vi "Test Summary on Failing Case Result.vi"(8 "error in (no error)":errorcluster, 11 "Result Model Result Recording Test in":refnum<class "Result Model Result Recording Test.lvclass">) -> (0 "error out":errorcluster, 3 "Result Model Result Recording Test out":refnum<class "Result Model Result Recording Test.lvclass">)   [LabVIEW 2020, in "Result Model Result Recording Test.lvclass"]
uses:
  Result Model Result Recording Test.lvclass
  Result Model Result Recording Test.lvclass/Result Model Result Recording Test.ctl
  source/Core/Result/Type.ctl
  source/Core/Result/Result.lvlib
  source/Core/Result/Status.ctl
  source/Core/Result/Result.ctl
  source/User Interface/Result Model/Result Model.lvclass
  ae2c71b8-32bb-49d1-8500-0119bfec74ff.vi
  C:/git/astemes-lunit/source/User Interface/Result Model/Result Model.lvclass
  C:/git/astemes-lunit/source/Framework/Result Observer/Result Observer.lvclass
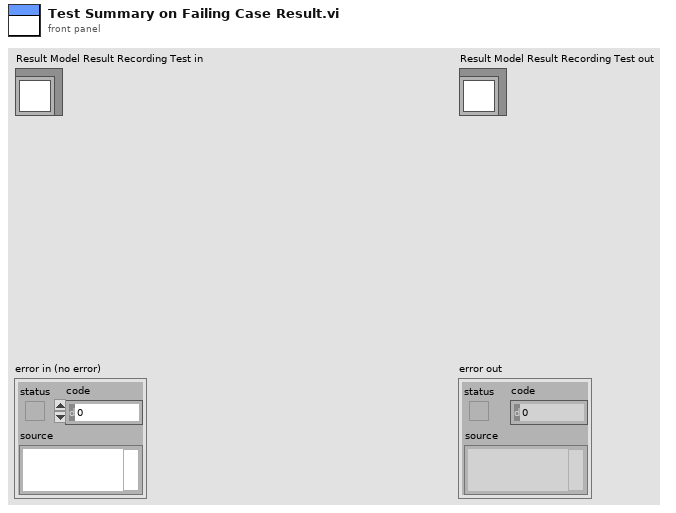
[diagram p1: front panel]
types:
  T1 = typedef "Result.lvlib/Result.ctl" = cluster{"Name":string, "Message":string, "Description":string, "Status":T2, "Result Type":T3, "Execution Time":dbl}
  T2 = typedef "Result.lvlib/Status.ctl" = enum16{"", "Passed", "Failed", "Error", "Skipped", "Setup Error", "Broken", "Teardown Error"}
  T3 = typedef "Result.lvlib/Type.ctl" = enum16{"Method", "Case", "Suite", "Pass", "Fail", "Skip", "Pass if", "Fail if", "Pass if Error", "Fail if Error", "Pass if Equal", "Fail if Equal"}
  T4 = cluster{"Left Cell String":string, "Child Text":string[], "Child Tag":string, "Item Indent":i32, "Child Only?":bool, "Glyph Index":i32}[]
  T5 = cluster{"Left Cell String":string, "Child Text":string[], "Child Tag":string, "Item Indent":i32, "Child Only?":bool, "Glyph Index":i32}
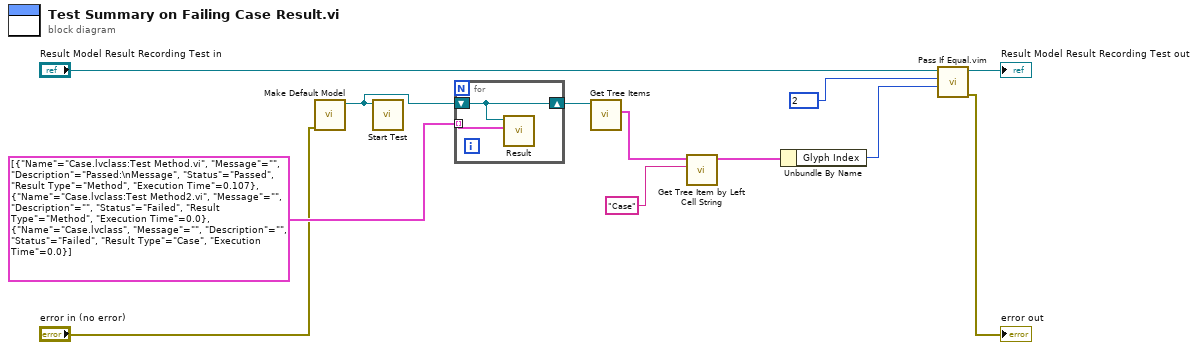
[diagram p0: block diagram]
diagram:
  n1 = call "Make Default Model.vi"("error in (no error)"="error in (no error)") -> ("Result Model out"=w1:refnum<class "Result Model.lvclass">)  [unwired: 9 in, 1 out]
  n2 = call "Start Test.vi"("Result Model In"=w1) -> ()  [unwired: 10 in, 1 out]
  n3 = for {
    tunnel: T1[] [{"Name"="Case.lvclass:Test Method.vi", "Message"="", "Description"="Passed:\nMessage", "Status"=enum."Passed", "Result Type"=enum."Method", "Execution Time"=0.107}, {"Name"="Case.lvclass:Test Method2.vi", "Message"="", "Description"="", "Status"=enum."Failed", "Result Type"=enum."Method", "Execution Time"=0.0}, {"Name"="Case.lvclass", "Message"="", "Description"="", "Status"=enum."Failed", "Result Type"=enum."Case", "Execution Time"=0.0}] ("Results") -> [w14] mode=indexing
    shift-right: [w13] -> w11
    shift-left: w1 -> [w13]
    n4 = call-dynamic "Result.vi"("Results"=w14, "Result Model in"=w13) -> ()  [unwired: 9 in, 1 out]
  }
  n5 = call "Get Tree Items.vi"("Result Model In"=w11) -> ("Tree Items"=w10:T4)  [unwired: 9 in, 1 out]
  n6 = call "Get Tree Item by Left Cell String.vi"("Left Cell String"="Case", "Tree Items"=w10) -> ("Item"=w6:T5)  [unwired: 9 in]
  n7 = Unbundle By Name(w6) -> ("Glyph Index"=w5:i32)
  n8 = call "Pass If Equal.vim"("Actual"=w5, "Expected"=2 ("Listbox Symbol Ring Constant"), "LUnit Test Case In"="Result Model Result Recording Test in") -> ("error out"=→"error out":errorcluster, "LUnit Test Case Out"=→"Result Model Result Recording Test out":refnum<class "Result Model Result Recording Test.lvclass">)  [unwired: 7 in]
